vi "Fields Get New Custom Field ID.vi"(3 "Existing Field IDs (empty)":string[](array[string])) -> (1 "Custom Field ID":string)   [LabVIEW 2011]
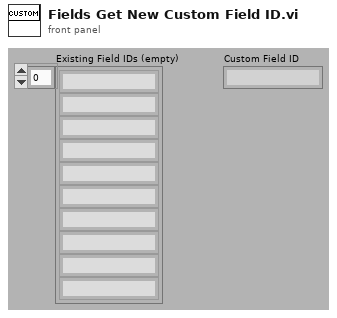
[diagram p1: front panel]
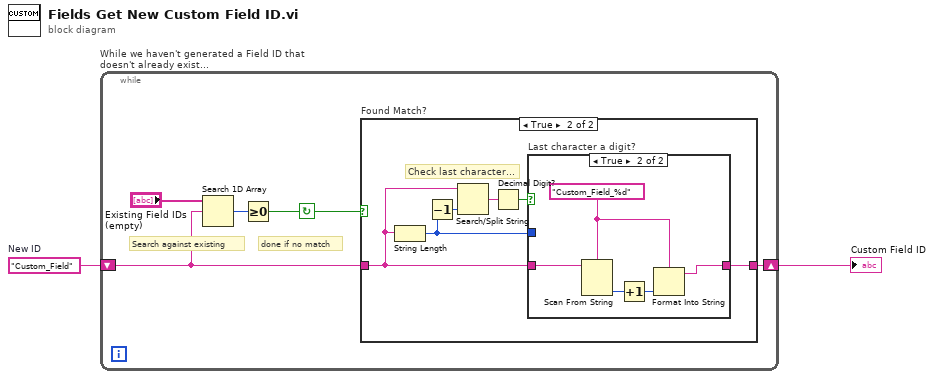
[diagram p0: block diagram]
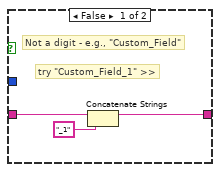
[diagram p3: hidden frame]
diagram:
  w1 = "Custom_Field"  # New ID
  n1 = while "While we haven't generated a Field ID that doesn't already exist..." {
    shift-right: [w6] -> w2
    shift-left: w1 -> [w5]
    stop <- w3 continue-if-true
    # "done if no match"
    # "Search against existing"
    n2 = Search 1D Array(1D array="Existing Field IDs (empty)", element=w5) -> (index of element=w7:i32)  [unwired: 1 out]
    n3 = Greater Or Equal To 0?(x=w7) -> (x >= 0?=w3:bool)
    n4 = case "Found Match?" shown="True" w3 {
      tunnel: w5 -> [w8 w10]
      tunnel: [w8 w14] -> w6
      frame False {
        # "No match - pass out current ID"
      }
      frame True {
        # "Check last character..."
        n5 = String Length(string=w10) -> (length=w9:i32)
        n6 = Decrement(x=w9) -> (x-1=w13:i32)
        n7 = Search/Split String(string=w10, offset (0)=w13) -> (match + rest of string=w11:string)  [unwired: 3 out]
        n8 = Decimal Digit?(1:w11) -> (0:w12:bool)
        n9 = case "Last character a digit?" shown="True" w12 {
          tunnel: [w17 w22] -> w14
          tunnel: w10 -> [w15 w18]
          tunnel: w9 -> [_ _]
          frame False {
            # "try \"Custom_Field_1\" >>"
            # "Not a digit - e.g., \"Custom_Field\""
            n10 = Concatenate Strings(w15, "_1") -> (w17:string)
          }
          frame True {
            w19 = "Custom_Field_%d"
            n11 = Scan From String(format string=w19, input string=w18) -> (output 1=w20:i32)  [unwired: 2 in, 4 out]
            n12 = Increment(x=w20) -> (x+1=w21:i32)
            n13 = Format Into String(format string=w19, w21) -> (resulting string=w22:string)  [unwired: 2 in, 1 out]
          }
        }
      }
    }
  }
  "Custom Field ID" <- w2
